vi "Parse End Label.vi"(8 "error in (no error)":errorcluster, 11 "Alpaca CLI Parser in":refnum<class "JSON Parser.lvclass">) -> (0 "error out":errorcluster, 3 "Alpaca CLI Parser out":refnum<class "JSON Parser.lvclass">)   [LabVIEW 2013, in "JKI JSON Serialization.lvlib" / "JSON Parser.lvclass"]
uses:
  JSON Parser.lvclass
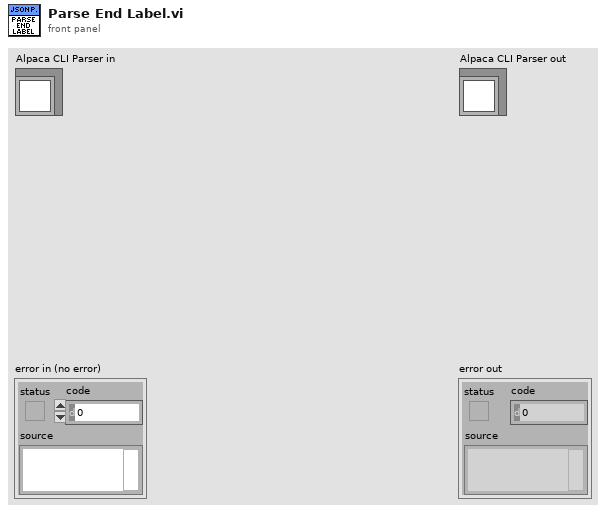
[diagram p1: front panel]
types:
  T1 = typedef "JKI JSON Serialization.lvlib/JSON Lexer.lvclass/JSON Token Type.ctl" = enum32{"unknown", "comma", "end-label", "begin-object", "end-object", "begin-array", "end-array", "quoted-string", "boolean", "exponential-number", "decimal-number", "integer-number", "special-number", "null", "symbol", "whitespace", "EOF"}
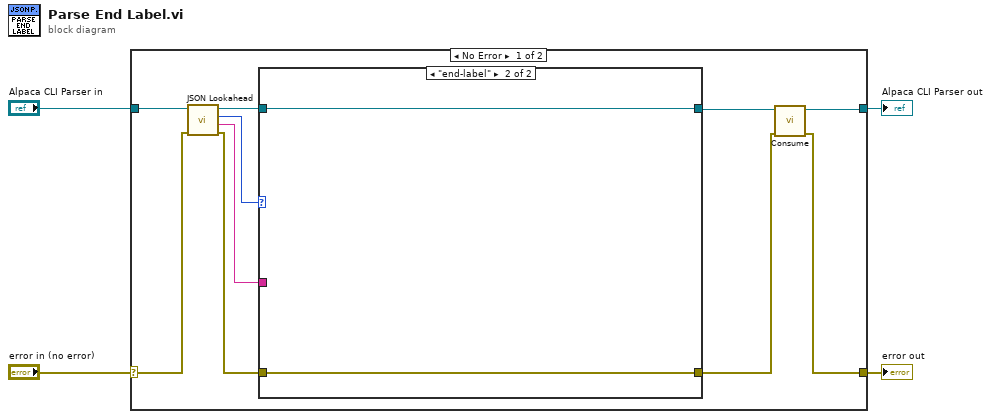
[diagram p0: block diagram]
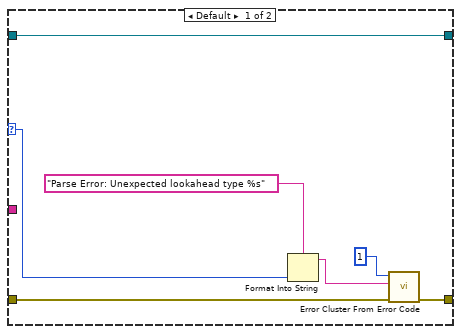
[diagram p2: hidden frame]
diagram:
  n1 = case shown="No Error" "error in (no error)" {
    selector: "error in (no error)" -> [w13 w25]
    tunnel: [w7 w25] -> w3
    tunnel: [w5 w24] -> w1
    tunnel: "Alpaca CLI Parser in" -> [w14 w24]
    frame No Error {
      n2 = call "JSON Lookahead.vi"("error in (no error)"=w13, "Alpaca CLI Parser in"=w14) -> ("error out"=w10:errorcluster, "Lookahead Value"=w9:string, "Lookahead Type"=w11:T1, "Alpaca CLI Parser out"=w12:refnum<class "JSON Parser.lvclass">)  [unwired: 6 in]
      n3 = case shown="\"end-label\"" w11 {
        selector: w11 -> [w17 _]
        tunnel: w12 -> [w15 w23]
        tunnel: [w15 w23] -> w8
        tunnel: [w21 w22] -> w6
        tunnel: w10 -> [w20 w22]
        tunnel: w9 -> [_ _]
        frame Default {
          n4 = Format Into String(format string="Parse Error: Unexpected lookahead type %s" ("error message (\"\")"), w17) -> (resulting string=w16:string)  [unwired: 2 in, 1 out]
          n5 = call <vilib>:"Error Cluster From Error Code.vi"("error in (no error)"=w20, "error message (\"\")"=w16, "error code (0)"=1) -> ("error out"=w21:errorcluster)  [unwired: 6 in]
        }
        frame "end-label" {
        }
      }
      n6 = call-dynamic "Consume.vi"("error in (no error)"=w6, "Alpaca Parser in"=w8) -> ("error out"=w7:errorcluster, "Alpaca Parser out"=w5:refnum<class "JSON Parser.lvclass">)  [unwired: 8 in]
    }
    frame Error {
    }
  }
  "error out" <- w3
  "Alpaca CLI Parser out" <- w1
